vi "ConfigureSimulatedData.vi"() -> ()   [LabVIEW 2017, in "CmsAcquisition.lvlib"]
uses:
  <vilib>/addons/InsightCM/Devices/Shared/Cms/CmsAcquisition/CmsAcquisition.lvlib
  <vilib>/addons/InsightCM/Devices/Shared/Cms/CmsAcquisition/controls/AcqSimulated_SignalConfig.ctl
  <vilib>/addons/InsightCM/Devices/Shared/Cms/CmsAcquisition/controls/AcqSimulated_Channels.ctl
  <vilib>/addons/InsightCM/Devices/Shared/Cms/CmsAcquisition/controls/AcqSimulated_ConfigRefs.ctl
  <vilib>/addons/InsightCM/Devices/Shared/Cms/CmsAcquisition/subVIs/SimulatedConfigRefGlobal.vi
panel:
  in  "Rule":T1(ring)
  in  "Short":bool[](array[boolean])
  in  "Open":bool[](array[boolean])
  in  "signal config":T2={"SimChannels"={"Name"=[], "Vibration"=[]}, "DutyCycle (%)"=10.0, "Add Noise?"=TRUE, "NoiseAmplitude"=0.1, "Offset"=0.0, "SamplingInfo"={"Fs"=1000.0, "#s"=1000.0}, "TachMode1-Ch0"=FALSE, "Offsets"=[]} {"SamplingInfo"."Fs" format="%.2p"; "NoiseAmplitude" format="%.2f"}
  in  "tachometer":cluster{"RPM":sgl}={"RPM"=100.0} {"RPM" min=100 max=3800 step=10 scale=100.0..1300.0}
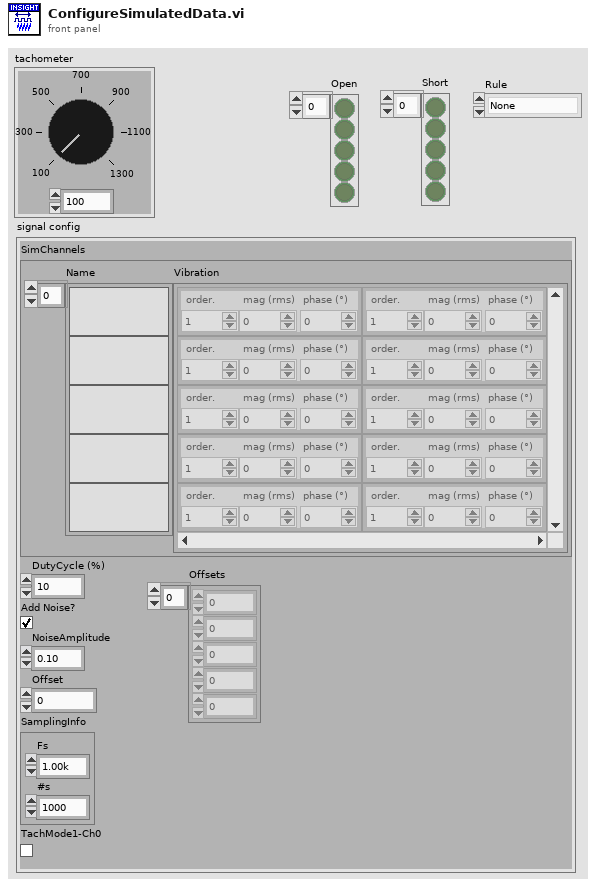
[diagram p1: front panel]
types:
  T1 = enum16{"None", "Pk_PkPK", "N Rule", "Z Rule", "U Rule", "Line Noise", "Low Signal", "Ski Slope", "Envelope Test"}
  T2 = typedef "CmsAcquisition.lvlib/AcqSimulated_SignalConfig.ctl" = cluster{"SimChannels":T3, "DutyCycle (%)":dbl, "Add Noise?":bool, "NoiseAmplitude":dbl, "Offset":dbl, "SamplingInfo":cluster{"Fs":dbl, "#s":dbl}, "TachMode1-Ch0":bool, "Offsets":dbl[]}
  T3 = typedef "CmsAcquisition.lvlib/AcqSimulated_Channels.ctl" = cluster{"Name":string[], "Vibration":cluster{"order.":dbl, "mag (rms)":dbl, "phase (°)":dbl}[][]}
  T4 = typedef "CmsAcquisition.lvlib/AcqSimulated_ConfigRefs.ctl" = cluster{"SignalConfigReference":refnum<vi>, "TachometerConfigReference":refnum<vi>}
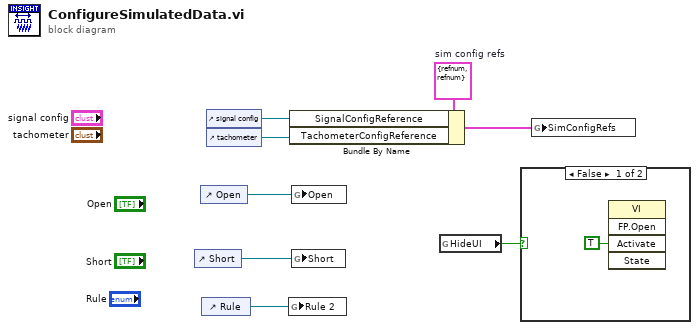
[diagram p0: block diagram]
diagram:
  w8 = T4 {"SignalConfigReference"=refnum, "TachometerConfigReference"=refnum}  # sim config refs
  n1 = control-ref of="Short"() -> (w3:refnum<vi>)
  n2 = control-ref of="Open"() -> (w4:refnum<vi>)
  n3 = control-ref of="Rule"() -> (w2:refnum<vi>)
  n4 = control-ref of="signal config"() -> (w7:refnum<vi>)
  n5 = control-ref of="tachometer"() -> (w6:refnum<vi>)
  n6 = global write "SimulatedConfigRefGlobal.vi" "Rule 2"(w2) -> ()
  n7 = Bundle By Name(cluster=w8, "SignalConfigReference"=w7, "TachometerConfigReference"=w6) -> (w5:T4)
  n8 = global write "SimulatedConfigRefGlobal.vi" "Open"(w4) -> ()
  n9 = global write "SimulatedConfigRefGlobal.vi" "Short"(w3) -> ()
  n10 = global read "SimulatedConfigRefGlobal.vi" "HideUI"() -> (w1:bool)
  n11 = case shown="False" w1 {
    frame False {
      n12 = invoke class="VI" method="FP.Open"("Activate"=TRUE ("Activate?")) -> ()  [unwired: 4 in, 5 out]
    }
    frame True {
    }
  }
  n13 = global write "SimulatedConfigRefGlobal.vi" "SimConfigRefs"(w5) -> ()
